vi "lidar_packages.vi"(3 "error in":errorcluster, 5 "Settings":T1) -> (0 "error out":errorcluster, 1 "Number points":i32, 2 "Packets":i32)   [LabVIEW 2025]
doc: "Calculate how many packages to send thu UDP based on the LiDAR configuration."
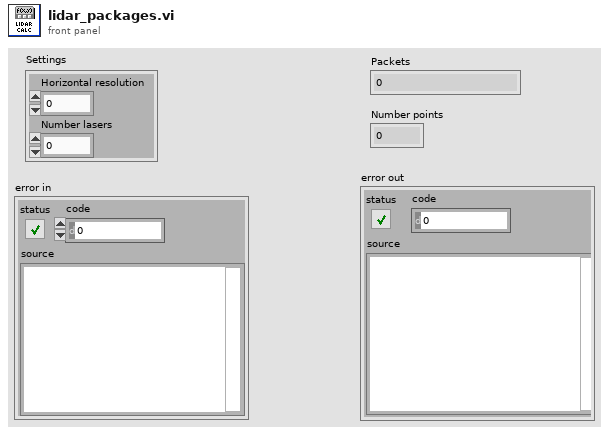
[diagram p1: front panel]
types:
  T1 = cluster{"Horizontal resolution":dbl, "Number lasers":i32}
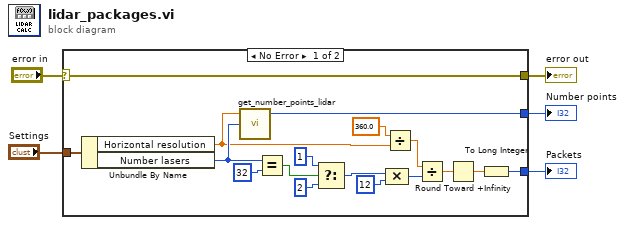
[diagram p0: block diagram]
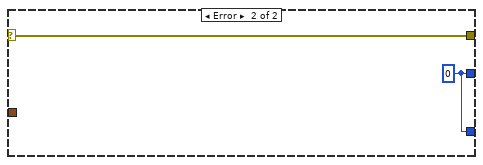
[diagram p2: hidden frame]
diagram:
  n1 = case shown="No Error" "error in" {
    selector: "error in" -> [w19 w24]
    tunnel: "Settings" -> [w22 _]
    tunnel: [w19 w24] -> w3
    tunnel: [w14 w23] -> w2
    tunnel: [w13 w23] -> w1
    frame No Error {
      n2 = Unbundle By Name(w22) -> ("Horizontal resolution"=w10:dbl, "Number lasers"=w11:i32)
      n3 = call "get_number_points_lidar.vi"("Number lasers"=w11, "Horizontal_resolution"=w10) -> ("Number points"=w13:i32)  [unwired: 3 in]
      n4 = Equal?(x=w11, y=32) -> (x = y?=w17:bool)
      n5 = Select(t=1, s=w17, f=2 ("t")) -> (s? t:f=w12:i32)
      n6 = Divide(x=360.0, y=w10) -> (x/y=w8:dbl)
      n7 = Compound Arithmetic op=MULTIPLY(w12, 12 ("value")) -> (w9:i32)
      n8 = Divide(x=w8, y=w9) -> (x/y=w7:dbl)
      n9 = Round Toward +Infinity(x=w7) -> (ceil(x): smallest int >= x=w6:dbl)
      n10 = To Long Integer(number=w6) -> (32bit integer=w14:i32)
    }
    frame Error {
      w23 = 0
    }
  }
  "error out" <- w3
  "Packets" <- w2
  "Number points" <- w1
